vi "ChannelControl.vi"() -> ()   [LabVIEW 2011]
uses:
  Global/Globalclient.vi
panel:
  out "选中行":i32
  out "删除通道":string[](array[string])
  in  "Stop Button":bool
  in  "通道":i32[](listbox)
  in  "Tab":enum32{"RF", "CLK"}(tab)
  in  "查询差损":bool
  in  "释放通道":bool
  in  "申请通道":bool
  out "LOSS":cluster{dbl[], dbl[]}[](graph)
  out "开关信息":string
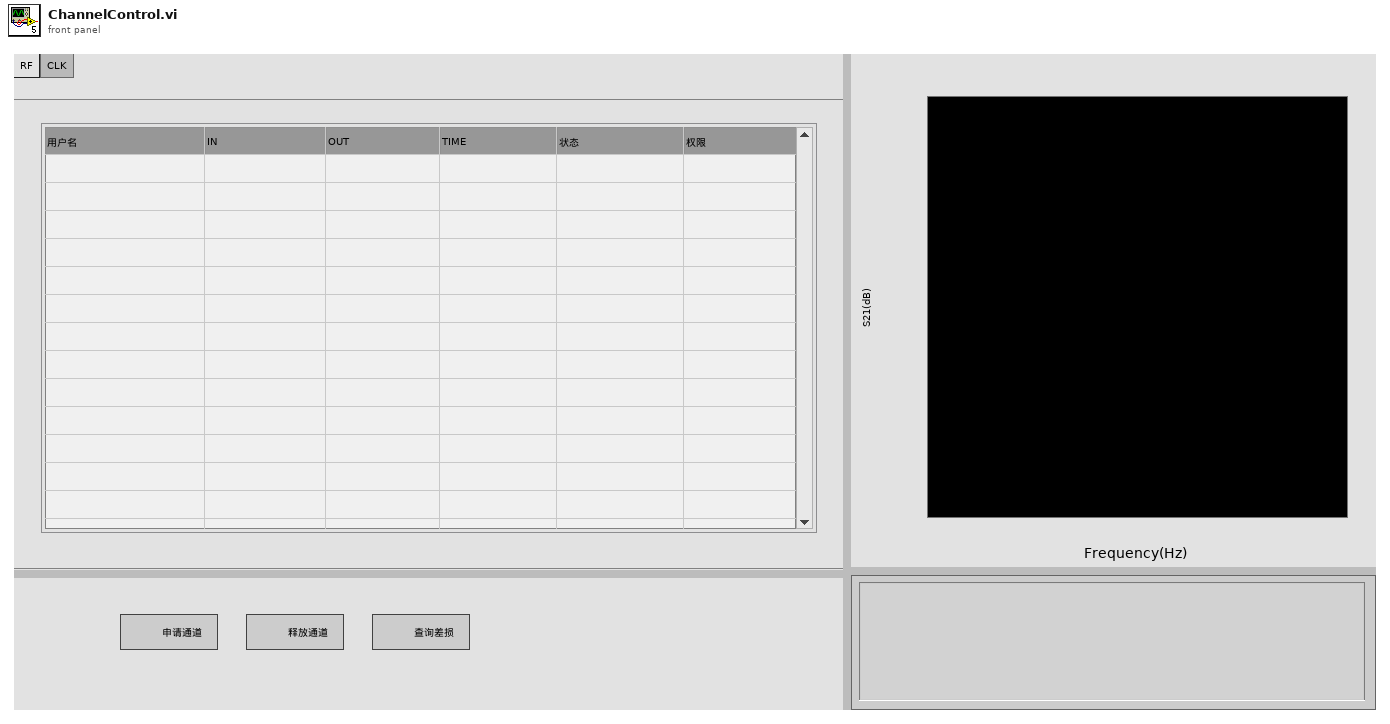
[diagram p1: front panel]
types:
  T1 = enum16{"Standard", "Buffered", "CRLF", "Immediate"}
  T2 = typedef "LVPoint32TypeDef.ctl" = cluster{"Horizontal":i32, "Vertical":i32}
  T3 = typedef "LVRowAndColumnTypeDef.ctl" = cluster{"Row":i32, "Column":i32}
  T4 = cluster{"data name":string, "data data":string}[]
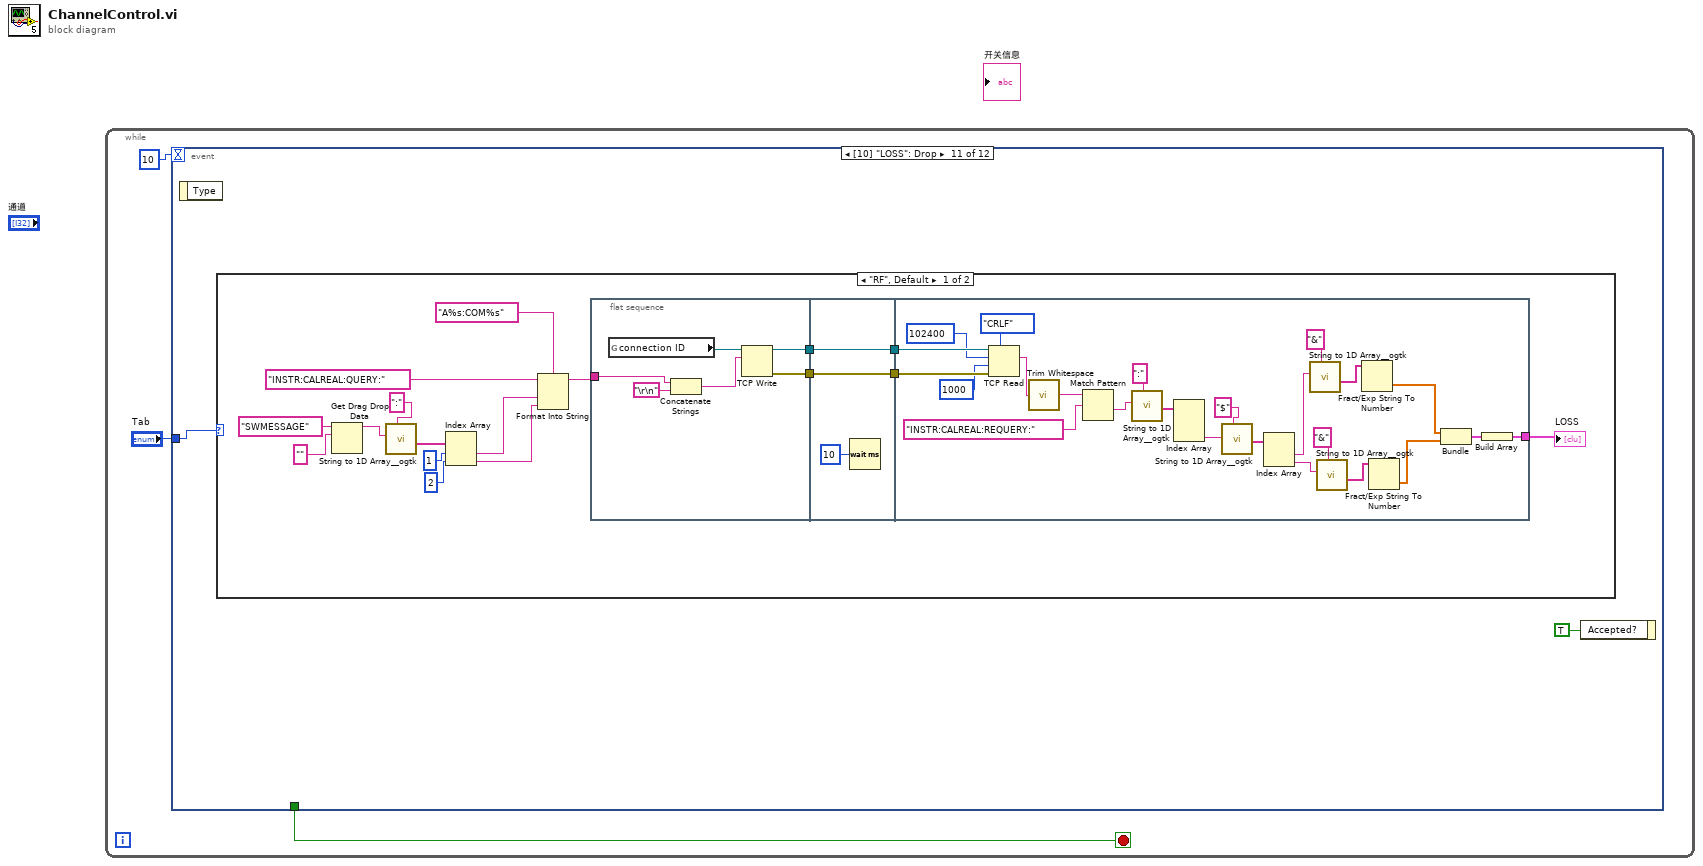
[diagram p0: block diagram]
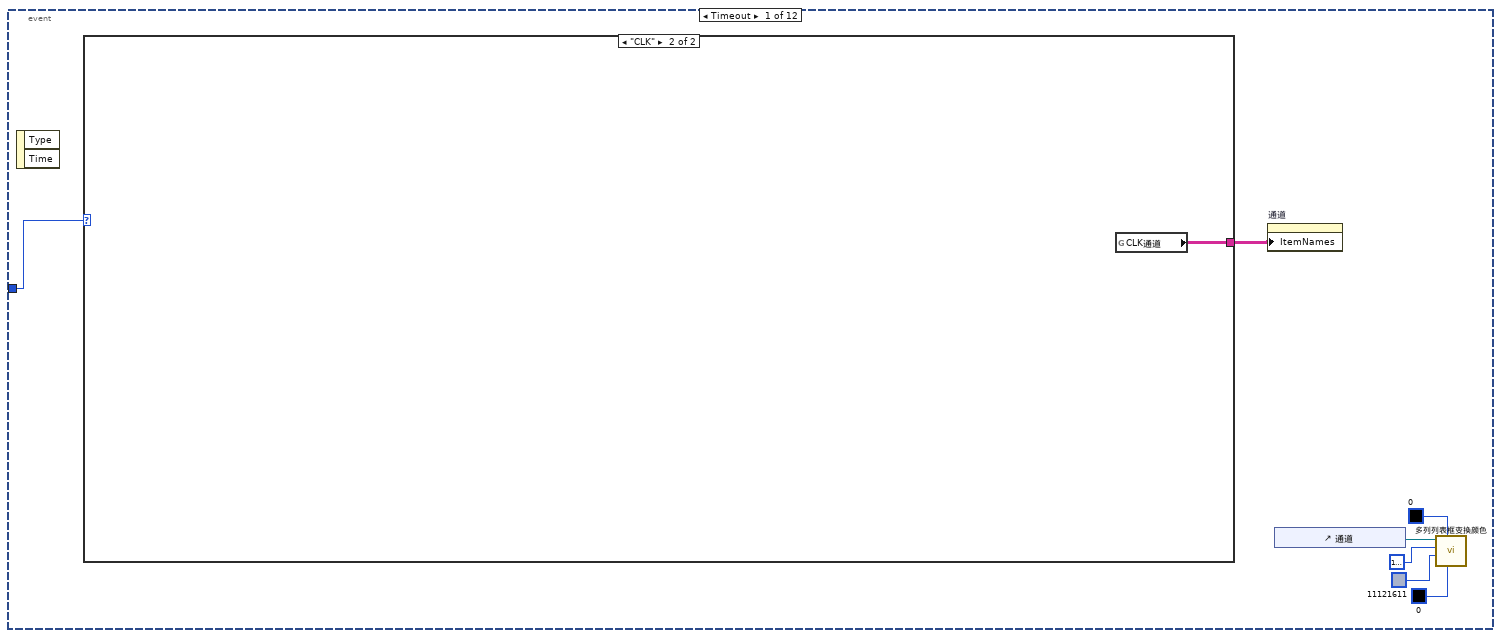
[diagram p2: hidden frame]
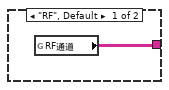
[diagram p3: hidden frame]
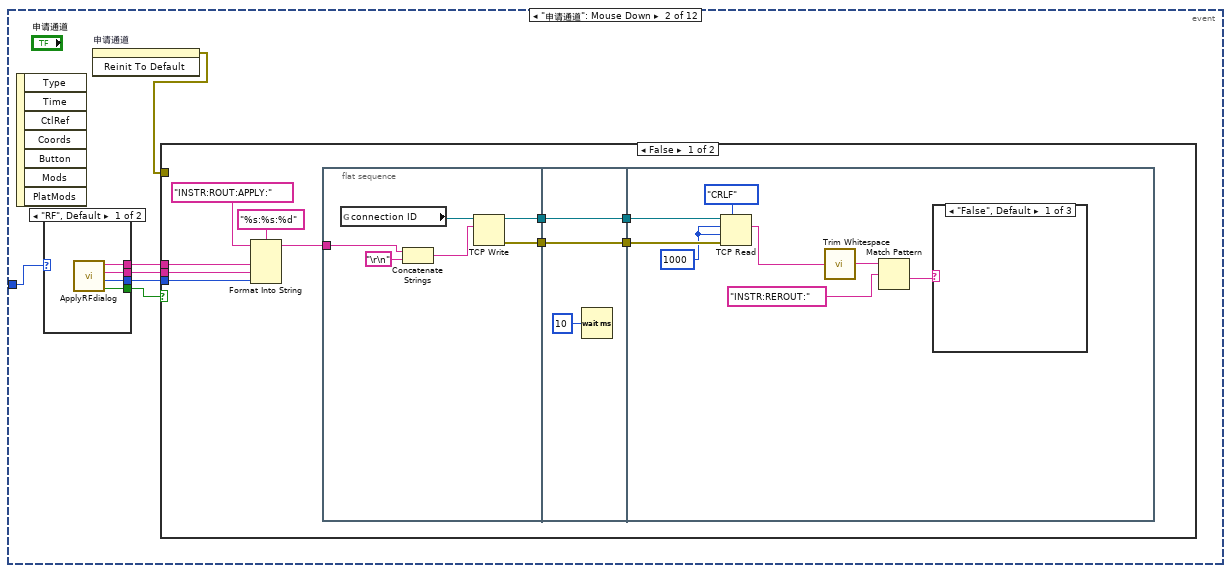
[diagram p4: hidden frame]
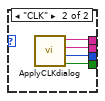
[diagram p5: hidden frame]
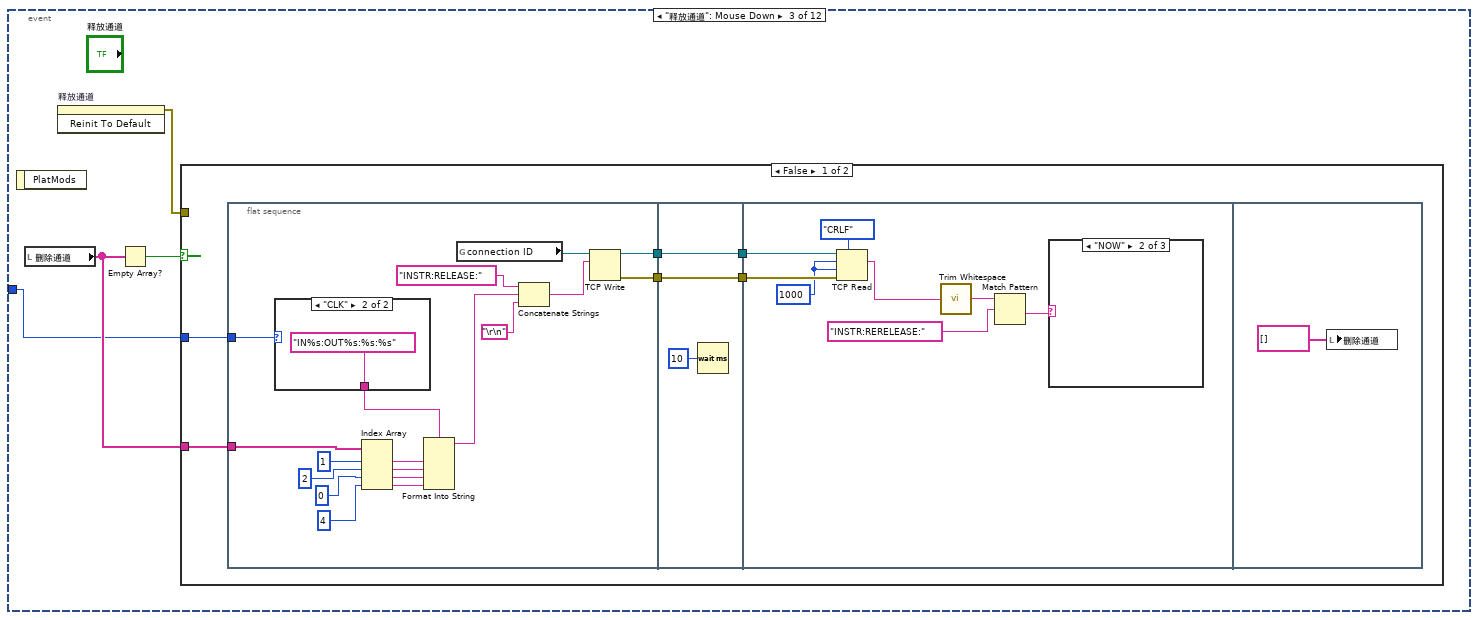
[diagram p9: hidden frame]
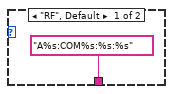
[diagram p10: hidden frame]
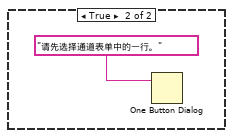
[diagram p13: hidden frame]
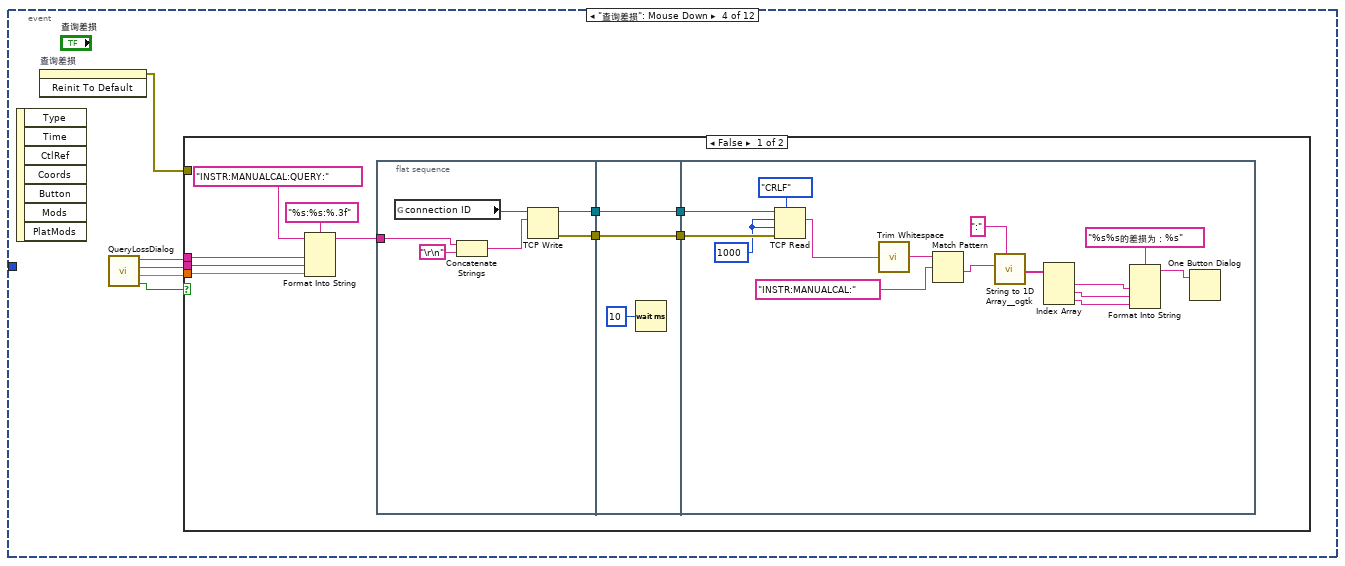
[diagram p14: hidden frame]
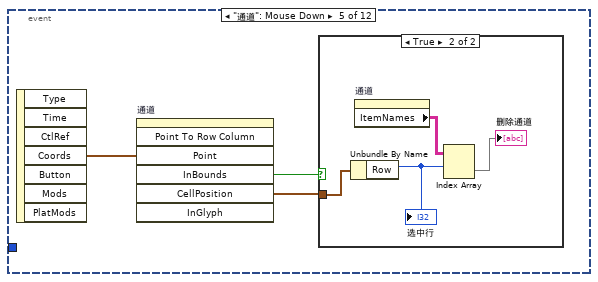
[diagram p16: hidden frame]
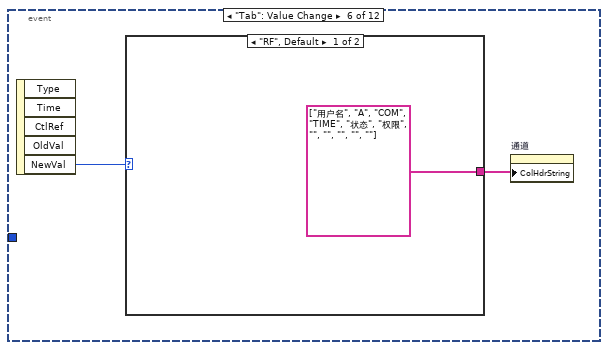
[diagram p18: hidden frame]
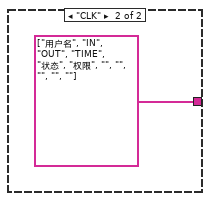
[diagram p19: hidden frame]
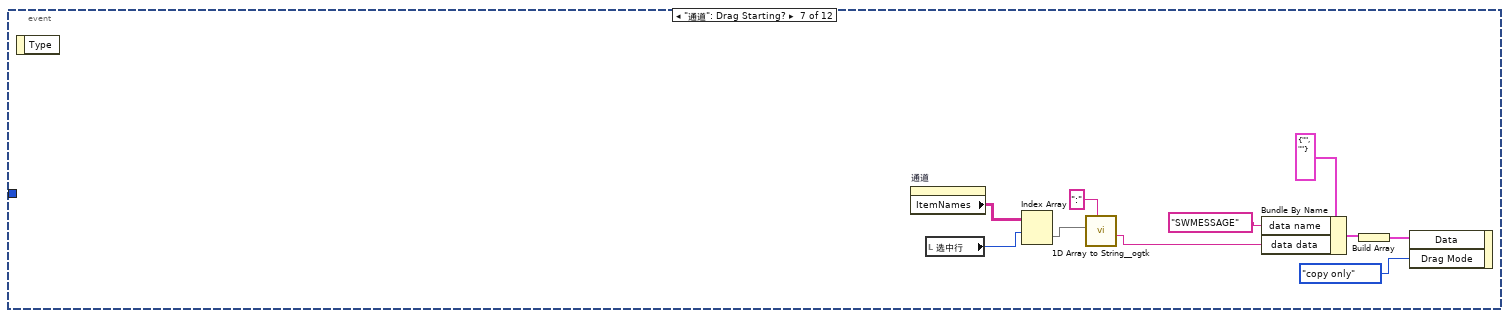
[diagram p20: hidden frame]
diagram:
  n1 = while {
    stop <- w3 stop-if-true
    n2 = event shown="[10] \"LOSS\": Drop" {
      selector: _ -> [_ _ _ _ _ _ _ _ _ _ _ _]
      dyn-events: _ -> [_ _ _ _ _ _ _ _ _ _ _ _]
      timeout: 10 -> [_ _ _ _ _ _ _ _ _ _ _ _]
      tunnel: [_ _ _ _ _ _ _ _ _ _ _ w219] -> w3
      tunnel: "Tab" -> [w10 w14 w55 _ _ _ _ _ _ _ w167 _]
      event Timeout {
        n3 = event-data() -> ()  [unwired: 1 in, 2 out]
        n4 = case shown="\"CLK\"" w10 {
          tunnel: [w11 w12] -> w9
          frame "RF", Default {
            n5 = global read "Globalclient.vi" "RF通道"() -> (w11:string[][])
          }
          frame "CLK" {
            n6 = global read "Globalclient.vi" "CLK通道"() -> (w12:string[][])
          }
        }
        n7 = property on="通道" class="MCListbox (strict)"("ItemNames"=w9) -> ()  [unwired: 2 in, 2 out]
        n8 = control-ref of="通道"() -> (w4:refnum<vi>)
        n9 = call "多列列表框变换颜色.vi"("奇数行字体颜色"=u32 0, "偶数行字体颜色"=u32 0, "奇数行背景颜色"=u32 11121611, "偶数行背景颜色"=u32 16777238, "MCListbox Refnum in"=w4) -> ()  [unwired: 5 in, 2 out]
      }
      event "申请通道": Mouse Down {
        n10 = event-data() -> ()  [unwired: 1 in, 7 out]
        n11 = case shown="\"RF\", Default" w14 {
          tunnel: [w22 w23] -> w18
          tunnel: [w21 w26] -> w17
          tunnel: [w20 w25] -> w16
          tunnel: [w19 w24] -> w15
          frame "RF", Default {
            n12 = call "ApplyRFdialog.vi"() -> ("drop?"=w22:bool, "时钟（分钟） 2"=w19:u32, "射频出 2"=w20:string, "射频进 2"=w21:string)  [unwired: 8 in]
          }
          frame "CLK" {
            n13 = call "ApplyCLKdialog.vi"() -> ("drop?"=w23:bool, "时间（分钟） 2"=w24:u32, "时钟出 2"=w25:string, "时钟进 2"=w26:string)  [unwired: 8 in]
          }
        }
        n14 = invoke on="申请通道" class="Bool" method="Reinit To Default"() -> (error out=w13:errorcluster)  [unwired: 3 in, 2 out]
        n15 = case shown="False" w18 {
          tunnel: w17 -> [w30 _]
          tunnel: w16 -> [w29 _]
          tunnel: w15 -> [w28 _]
          tunnel: w13 -> [_ _]
          frame False {
            n16 = Format Into String(format string="%s:%s:%d", initial string="INSTR:ROUT:APPLY:", w30, w29, w28) -> (resulting string=w27:string)  [unwired: 1 in, 1 out]
            n17 = flat-sequence {
              tunnel: [w39] -> w36
              tunnel: [w38] -> w35
              tunnel: w27 -> [w37]
              tunnel: [w45] -> w34
              tunnel: w36 -> [w45]
              tunnel: [w44] -> w33
              tunnel: w35 -> [w44]
              tunnel: w34 -> [w53]
              tunnel: w33 -> [w52]
              frame #0 {
                n18 = global read "Globalclient.vi" "connection ID"() -> (w42:refnum<k5>)
                n19 = Concatenate Strings(w37, "\r\n") -> (w40:string)
                n20 = TCP Write(connection ID=w42, data in=w40) -> (connection ID out=w39:refnum<k5>, error out=w38:errorcluster)  [unwired: 2 in, 1 out]
              }
              frame #1 {
                n21 = Wait (ms)(milliseconds to wait=u32 10) -> ()  [unwired: 1 out]
              }
              frame #2 {
                w50 = 1000
                n22 = TCP Read(connection ID=w53, bytes to read=w50, error in (no error)=w52, 7:T1."CRLF" ("mode (standard)"), 9:w50) -> (data out=w49:string)  [unwired: 2 out]
                n23 = call <vilib>:"Trim Whitespace.vi"("string"=w49) -> ("trimmed string"=w48:string)  [unwired: 1 in]
                n24 = Match Pattern(string=w48, regular expression="INSTR:REROUT:") -> (after substring=w46:string)  [unwired: 1 in, 3 out]
                n25 = case shown="\"False\", Default" w46 {
                  frame "False", Default {
                  }
                  frame "NOW" {
                  }
                  frame "WAIT" {
                  }
                }
              }
            }
          }
          frame True {
          }
        }
      }
      event "释放通道": Mouse Down {
        n26 = event-data() -> ()  [unwired: 1 in, 1 out]
        n27 = local read "删除通道"() -> (w56:string[])
        n28 = invoke on="释放通道" class="Bool" method="Reinit To Default"() -> (error out=w54:errorcluster)  [unwired: 3 in, 2 out]
        n29 = Empty Array?(array=w56) -> (empty?=w57:bool)
        n30 = case shown="False" w57 {
          tunnel: w56 -> [w59 _]
          tunnel: w55 -> [w58 _]
          tunnel: w54 -> [_ _]
          frame False {
            n31 = flat-sequence {
              tunnel: [w78] -> w63
              tunnel: [w77] -> w62
              tunnel: w59 -> [w71]
              tunnel: w58 -> [w64]
              tunnel: [w86] -> w61
              tunnel: w63 -> [w86]
              tunnel: [w85] -> w60
              tunnel: w62 -> [w85]
              tunnel: w61 -> [w94]
              tunnel: w60 -> [w93]
              frame #0 {
                n32 = case shown="\"CLK\"" w64 {
                  tunnel: ["A%s:COM%s:%s:%s" ("format string") "IN%s:OUT%s:%s:%s" ("format string")] -> w66
                  frame "RF", Default {
                  }
                  frame "CLK" {
                  }
                }
                n33 = Index Array(array=w71, index #1=1 ("index"), index #2=2 ("index"), index #3=0 ("index"), index #4=4 ("index")) -> (element #1=w70:string, element #2=w69:string, element #3=w68:string, element #4=w67:string)
                n34 = Format Into String(format string=w66, w70, w69, w68, w67) -> (resulting string=w65:string)  [unwired: 2 in, 1 out]
                n35 = global read "Globalclient.vi" "connection ID"() -> (w81:refnum<k5>)
                n36 = Concatenate Strings("INSTR:RELEASE:", w65, "\r\n") -> (w79:string)
                n37 = TCP Write(connection ID=w81, data in=w79) -> (connection ID out=w78:refnum<k5>, error out=w77:errorcluster)  [unwired: 2 in, 1 out]
              }
              frame #1 {
                n38 = Wait (ms)(milliseconds to wait=u32 10) -> ()  [unwired: 1 out]
              }
              frame #2 {
                w91 = 1000
                n39 = TCP Read(connection ID=w94, bytes to read=w91, error in (no error)=w93, 7:T1."CRLF" ("mode (standard)"), 9:w91) -> (data out=w90:string)  [unwired: 2 out]
                n40 = call <vilib>:"Trim Whitespace.vi"("string"=w90) -> ("trimmed string"=w89:string)  [unwired: 1 in]
                n41 = Match Pattern(string=w89, regular expression="INSTR:RERELEASE:") -> (after substring=w87:string)  [unwired: 1 in, 3 out]
                n42 = case shown="\"NOW\"" w87 {
                  frame "False", Default {
                  }
                  frame "NOW" {
                  }
                  frame "WAIT" {
                  }
                }
              }
              frame #3 {
                n43 = local write "删除通道"(string[] [] ("删除通道")) -> ()
              }
            }
          }
          frame True {
            n44 = One Button Dialog(message="请先选择通道表单中的一行。") -> ()  [unwired: 1 in, 1 out]
          }
        }
      }
      event "查询差损": Mouse Down {
        n45 = event-data() -> ()  [unwired: 1 in, 7 out]
        n46 = invoke on="查询差损" class="Bool" method="Reinit To Default"() -> (error out=w97:errorcluster)  [unwired: 3 in, 2 out]
        n47 = call "QueryLossDialog.vi"() -> ("drop?"=w98:bool, "频率（KHz） 2"=w99:dbl, "射频出 2"=w100:string, "射频进 2"=w101:string)  [unwired: 8 in]
        n48 = case shown="False" w98 {
          tunnel: w101 -> [w106 _]
          tunnel: w100 -> [w105 _]
          tunnel: w99 -> [w104 _]
          tunnel: w97 -> [_ _]
          frame False {
            n49 = Format Into String(format string="%s:%s:%.3f", initial string="INSTR:MANUALCAL:QUERY:", w106, w105, w104) -> (resulting string=w103:string)  [unwired: 1 in, 1 out]
            n50 = flat-sequence {
              tunnel: [w114] -> w111
              tunnel: [w113] -> w110
              tunnel: w103 -> [w112]
              tunnel: [w120] -> w109
              tunnel: w111 -> [w120]
              tunnel: [w119] -> w108
              tunnel: w110 -> [w119]
              tunnel: w109 -> [w135]
              tunnel: w108 -> [w134]
              frame #0 {
                n51 = global read "Globalclient.vi" "connection ID"() -> (w117:refnum<k5>)
                n52 = Concatenate Strings(w112, "\r\n") -> (w115:string)
                n53 = TCP Write(connection ID=w117, data in=w115) -> (connection ID out=w114:refnum<k5>, error out=w113:errorcluster)  [unwired: 2 in, 1 out]
              }
              frame #1 {
                n54 = Wait (ms)(milliseconds to wait=u32 10) -> ()  [unwired: 1 out]
              }
              frame #2 {
                w132 = 1000
                n55 = TCP Read(connection ID=w135, bytes to read=w132, error in (no error)=w134, 7:T1."CRLF" ("mode (standard)"), 9:w132) -> (data out=w131:string)  [unwired: 2 out]
                n56 = call <vilib>:"Trim Whitespace.vi"("string"=w131) -> ("trimmed string"=w130:string)  [unwired: 1 in]
                n57 = Match Pattern(string=w130, regular expression="INSTR:MANUALCAL:") -> (after substring=w128:string)  [unwired: 1 in, 3 out]
                n58 = call <userlib>:"String to 1D Array__ogtk.vi"("delimiter (Tab)"=":", "string"=w128) -> ("Array of Strings"=w126:string[])  [unwired: 9 in]
                n59 = Index Array(array=w126) -> (element #1=w124:string, element #2=w123:string, element #3=w122:string)  [unwired: 3 in]
                n60 = Format Into String(format string="%s%s的差损为：%s", w124, w123, w122) -> (resulting string=w121:string)  [unwired: 2 in, 1 out]
                n61 = One Button Dialog(message=w121) -> ()  [unwired: 1 in, 1 out]
              }
            }
          }
          frame True {
          }
        }
      }
      event "通道": Mouse Down {
        n62 = event-data() -> ("Coords"=w138:T2)  [unwired: 1 in, 6 out]
        n63 = invoke on="通道" class="MCListbox (strict)" method="Point To Row Column"("Point"=w138) -> ("InBounds"=w137:bool, "CellPosition"=w136:T3)  [unwired: 6 in, 5 out]
        n64 = case shown="True" w137 {
          tunnel: w136 -> [_ w142]
          frame False {
          }
          frame True {
            n65 = Unbundle By Name(w142) -> ("Row"=w141:i32)
            "选中行" <- w141
            n66 = property on="通道" class="MCListbox (strict)"() -> ("ItemNames"=w140:string[][])  [unwired: 2 in, 2 out]
            n67 = Index Array(array=w140, index (row)=w141) -> (element=→"删除通道":string[])  [unwired: 1 in]
          }
        }
      }
      event "Tab": Value Change {
        n68 = event-data() -> ("NewVal"=w144:enum32{"RF", "CLK"})  [unwired: 1 in, 4 out]
        n69 = case shown="\"RF\", Default" w144 {
          tunnel: [string[] ["用户名", "A", "COM", "TIME", "状态", "权限", "", "", "", "", ""] ("Column Header Strings[]") string[] ["用户名", "IN", "OUT", "TIME", "状态", "权限", "", "", "", "", ""] ("Column Header Strings[]")] -> w143
          frame "RF", Default {
          }
          frame "CLK" {
          }
        }
        n70 = property on="通道" class="MCListbox (strict)"("ColHdrString"=w143) -> ()  [unwired: 2 in, 2 out]
      }
      event "通道": Drag Starting? {
        n71 = event-data() -> ()  [unwired: 1 in, 1 out]
        n72 = property on="通道" class="MCListbox (strict)"() -> ("ItemNames"=w156:string[][])  [unwired: 2 in, 2 out]
        n73 = local read "选中行"() -> (w155:i32)
        n74 = Index Array(array=w156, index (row)=w155) -> (element=w153:string[])  [unwired: 1 in]
        n75 = call <userlib>:"1D Array to String__ogtk.vi"("delimiter (Tab)"=":", "Array of Strings"=w153) -> ("delimited string"=w149:string)  [unwired: 9 in]
        n76 = Bundle By Name(cluster=cluster{"data name":string, "data data":string} {"data name"="", "data data"=""}, "data name"="SWMESSAGE", "data data"=w149) -> (w152:cluster{"data name":string, "data data":string})
        n77 = Build Array(w152) -> (w148:T4)
        n78 = event-data("Data"=w148, "Drag Mode"=enum32{"copy or move", "copy only", "move only"}."copy only") -> ()  [unwired: 1 in, 1 out]
      }
      event "开关信息": Drag Enter {
        n79 = event-data() -> ()  [unwired: 1 in, 8 out]
        n80 = event-data("Accepted?"=TRUE) -> ()  [unwired: 1 in, 1 out]
      }
      event "开关信息": Drop {
        n81 = event-data() -> ()  [unwired: 1 in, 8 out]
        n82 = Get Drag Drop Data(8:"" ("type"), 9:"SWMESSAGE" ("data name")) -> (3:w161:string)  [unwired: 1 in, 1 out]
        n83 = call <userlib>:"String to 1D Array__ogtk.vi"("delimiter (Tab)"=":", "string"=w161) -> ("Array of Strings"=w162:string[])  [unwired: 9 in]
        n84 = Index Array(array=w162, index #1=1 ("index"), index #2=2 ("index")) -> ()  [unwired: 2 out]
        n85 = event-data("Accepted?"=TRUE) -> ()  [unwired: 1 in, 1 out]
      }
      event "LOSS": Drag Enter {
        n86 = event-data() -> ()  [unwired: 1 in, 8 out]
        n87 = event-data("Accepted?"=TRUE) -> ()  [unwired: 1 in, 1 out]
      }
      event "LOSS": Drop {
        n88 = event-data() -> ()  [unwired: 1 in, 1 out]
        n89 = case shown="\"RF\", Default" w167 {
          frame "RF", Default {
            n90 = Get Drag Drop Data(8:"" ("type"), 9:"SWMESSAGE" ("data name")) -> (3:w175:string)  [unwired: 1 in, 1 out]
            n91 = call <userlib>:"String to 1D Array__ogtk.vi"("delimiter (Tab)"=":", "string"=w175) -> ("Array of Strings"=w177:string[])  [unwired: 9 in]
            n92 = Index Array(array=w177, index #1=1 ("index"), index #2=2 ("index")) -> (element #1=w172:string, element #2=w171:string)
            n93 = Format Into String(format string="A%s:COM%s", initial string="INSTR:CALREAL:QUERY:", w172, w171) -> (resulting string=w170:string)  [unwired: 1 in, 1 out]
            n94 = flat-sequence {
              tunnel: [w188] -> w185
              tunnel: [w187] -> w184
              tunnel: w170 -> [w186]
              tunnel: [w194] -> w183
              tunnel: w185 -> [w194]
              tunnel: [w193] -> w182
              tunnel: w184 -> [w193]
              tunnel: w183 -> [w218]
              tunnel: w182 -> [w217]
              tunnel: [w207] -> w169
              frame #0 {
                n95 = global read "Globalclient.vi" "connection ID"() -> (w191:refnum<k5>)
                n96 = Concatenate Strings(w186, "\r\n") -> (w189:string)
                n97 = TCP Write(connection ID=w191, data in=w189) -> (connection ID out=w188:refnum<k5>, error out=w187:errorcluster)  [unwired: 2 in, 1 out]
              }
              frame #1 {
                n98 = Wait (ms)(milliseconds to wait=u32 10) -> ()  [unwired: 1 out]
              }
              frame #2 {
                n99 = TCP Read(connection ID=w218, bytes to read=102400, error in (no error)=w217, 7:T1."CRLF" ("mode (standard)"), 9:1000 ("timeout ms (25000)")) -> (data out=w214:string)  [unwired: 2 out]
                n100 = call <vilib>:"Trim Whitespace.vi"("string"=w214) -> ("trimmed string"=w213:string)  [unwired: 1 in]
                n101 = Match Pattern(string=w213, regular expression="INSTR:CALREAL:REQUERY:") -> (after substring=w209:string)  [unwired: 1 in, 3 out]
                n102 = call <userlib>:"String to 1D Array__ogtk.vi"("delimiter (Tab)"=":", "string"=w209) -> ("Array of Strings"=w210:string[])  [unwired: 9 in]
                n103 = Index Array(array=w210) -> (element #3=w205:string)  [unwired: 3 in, 2 out]
                n104 = call <userlib>:"String to 1D Array__ogtk.vi"("delimiter (Tab)"="$" ("search string"), "string"=w205) -> ("Array of Strings"=w203:string[])  [unwired: 9 in]
                n105 = Index Array(array=w203) -> (element #1=w202:string, element #2=w196:string)  [unwired: 2 in]
                n106 = call <userlib>:"String to 1D Array__ogtk.vi"("delimiter (Tab)"="&", "string"=w202) -> ("Array of Strings"=w200:string[])  [unwired: 9 in]
                n107 = call <userlib>:"String to 1D Array__ogtk.vi"("delimiter (Tab)"="&", "string"=w196) -> ("Array of Strings"=w198:string[])  [unwired: 9 in]
                n108 = Fract/Exp String To Number(string=w200) -> (number=w199:dbl[])  [unwired: 3 in, 1 out]
                n109 = Fract/Exp String To Number(string=w198) -> (number=w195:dbl[])  [unwired: 3 in, 1 out]
                n110 = Bundle(w199, w195) -> (w208:cluster{dbl[], dbl[]})  [unwired: 1 in]
                n111 = Build Array(w208) -> (w207:cluster{dbl[], dbl[]}[])
              }
            }
            "LOSS" <- w169
          }
          frame "CLK" {
          }
        }
        n112 = event-data("Accepted?"=TRUE) -> ()  [unwired: 1 in, 1 out]
      }
      event "Stop Button": Value Change {
        n113 = event-data() -> ("NewVal"=w219:bool)  [unwired: 1 in, 4 out]
      }
    }
  }
